vi "Send Data Packet.vi"(0 "connection ID":refnum<k5>, 5 "Packet #":u8, 7 "TCP/IP Data":u8[](array[numeric]), 9 "Timeout (15000ms)":i32=15000, 11 "error in":errorcluster) -> (4 "connection ID out":refnum<k5>, 15 "error out":errorcluster)   [LabVIEW 2014, in "hse-db.lvlib" / "MySQL (TCP).lvlib"]
uses:
  MySQL (TCP).lvlib
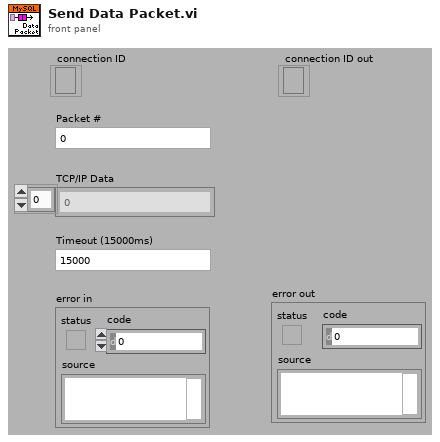
[diagram p1: front panel]
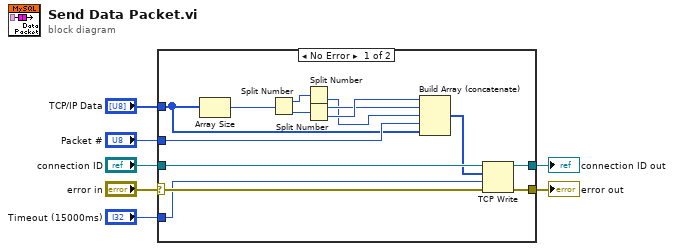
[diagram p0: block diagram]
diagram:
  n1 = case shown="No Error" "error in" {
    selector: "error in" -> [w9 w23]
    tunnel: "Timeout (15000ms)" -> [w8 _]
    tunnel: "connection ID" -> [w21 w22]
    tunnel: [w20 w23] -> w5
    tunnel: [w19 w22] -> w4
    tunnel: "Packet #" -> [w12 _]
    tunnel: "TCP/IP Data" -> [w11 _]
    frame No Error {
      n2 = Array Size(array=w11) -> (size(s)=w10:i32)
      n3 = Split Number(x=w10) -> (hi(x)=w18:u16, lo(x)=w17:u16)
      n4 = Split Number(x=w18) -> (lo(x)=w14:u8)  [unwired: 1 out]
      n5 = Split Number(x=w17) -> (hi(x)=w15:u8, lo(x)=w16:u8)
      n6 = Build Array (concatenate)(w16, w15, w14, w12, w11) -> (w13:u8[])
      n7 = TCP Write(connection ID=w21, data in=w13, error in (no error)=w9, 9:w8) -> (connection ID out=w19:refnum<k5>, error out=w20:errorcluster)  [unwired: 1 out]
    }
    frame Error {
    }
  }
  "connection ID out" <- w4
  "error out" <- w5
